vi "GL_heaterdisplay.vi"() -> ()   [LabVIEW 2024]
panel:
  out "Array":bool[](array[boolean])
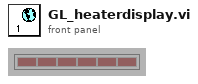
[diagram p1: front panel]
diagram:
